vi "Steuerung schreiben.vi"(8 "error in (no error)":errorcluster caption="Fehler (Eingang, kein Fehler)", 10 "Werte":T1, 11 "Steuerung PNS Eingang":refnum<class "Steuerung PNS.lvclass">) -> (0 "error out":errorcluster caption="Fehler (Ausgang)", 3 "Steuerung PNS Ausgang":refnum<class "Steuerung PNS.lvclass">)   [LabVIEW 2020, in "Steuerung PNS.lvclass"]
doc: "Low Level Schreiben auf die Steuerung der Werte vom Input.\nRIW"
uses:
  Steuerung PNS.lvclass
  Werte.ctl
  Steuerung PNS.lvclass/Steuerung PNS.ctl
  <vilib>/NI/Modbus Library/API/Master/Modbus Master.lvclass
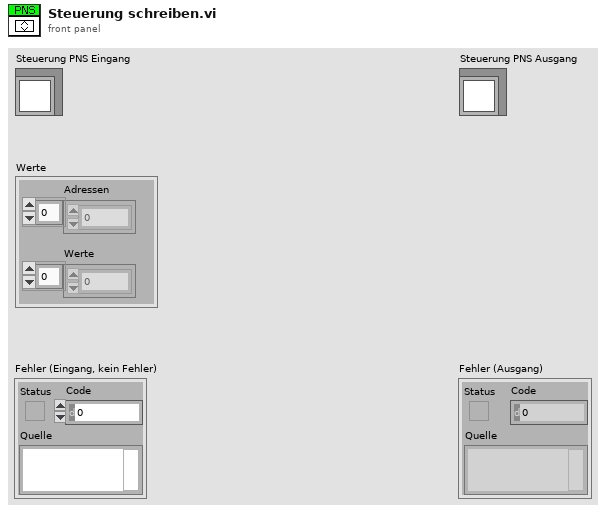
[diagram p1: front panel]
types:
  T1 = typedef "Steuerung PNS.lvclass/Werte.ctl" = cluster{"Adressen":u16[], "Werte":u16[]}
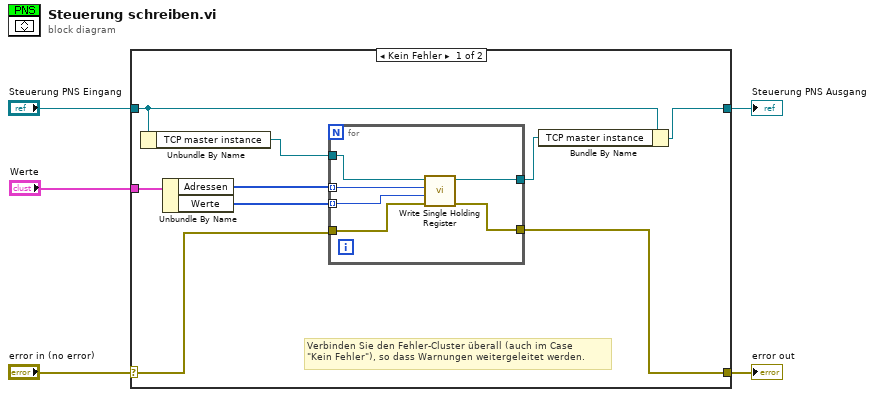
[diagram p0: block diagram]
diagram:
  n1 = case shown="Kein Fehler" "error in (no error)" {
    selector: "error in (no error)" -> [w14 w22]
    tunnel: [w13 w22] -> w4
    tunnel: [w10 w21] -> w2
    tunnel: "Steuerung PNS Eingang" -> [w11 w21]
    tunnel: "Werte" -> [w8 _]
    frame No Error {
      # "Verbinden Sie den Fehler-Cluster überall (auch im Case\n\"Kein Fehler\"), so dass Warnungen weitergeleitet werden."
      n2 = Unbundle By Name(w11) -> ("TCP master instance"=w12:refnum<class "Modbus Master.lvclass">)
      n3 = Unbundle By Name(w8) -> ("Adressen"=w7:u16[], "Werte"=w6:u16[])
      n4 = for {
        tunnel: w7 -> [w17] mode=indexing
        tunnel: [w20] -> w13
        tunnel: w14 -> [w19]
        tunnel: w6 -> [w18] mode=indexing
        tunnel: [w16] -> w9
        tunnel: w12 -> [w15]
        n5 = call-dynamic "Write Single Holding Register.vi"("error in"=w19, "register to write"=w18, "address"=w17, "Modbus master in"=w15) -> ("error out"=w20:errorcluster, "Modbus master out"=w16:refnum<class "Modbus Master.lvclass">)  [unwired: 6 in]
      }
      n6 = Bundle By Name(cluster=w11, "TCP master instance"=w9) -> (w10:refnum<class "Steuerung PNS.lvclass">)
    }
    frame Error {
    }
  }
  "error out" <- w4
  "Steuerung PNS Ausgang" <- w2
